vi "Execute.vi"(8 "error in":errorcluster, 11 "O3 Power On in":refnum<class "O3 Power On.lvclass">) -> (0 "error out":errorcluster, 1 "Next Step?":bool, 2 "MSG":string, 3 "O3 Power On out":refnum<class "O3 Power On.lvclass">)   [LabVIEW 2015, in "O3 Power On.lvclass"]
uses:
  O3 Power On.lvclass
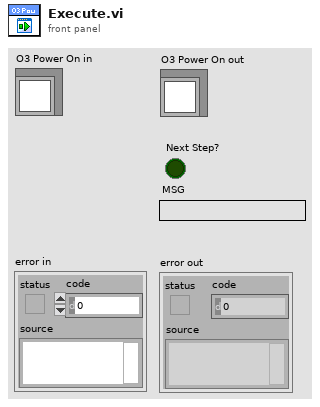
[diagram p1: front panel]
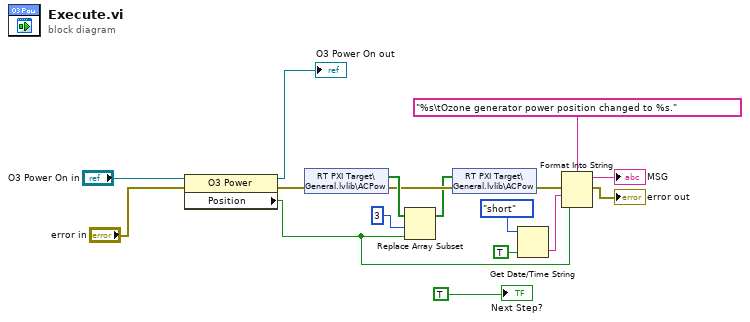
[diagram p0: block diagram]
diagram:
  n1 = property class="O3 Power"(reference="O3 Power On in", error in="error in") -> (reference out=→"O3 Power On out":refnum<class "O3 Power On.lvclass">, error out=w4:errorcluster, "Position"=w1:bool)
  n2 = shared-variable "RT PXI Target\\General.lvlib\\ACPow"(error in=w4) -> (w6:bool[], error out=w3:errorcluster)
  n3 = Replace Array Subset(array=w6, new element=w1, index=3) -> (w2:bool[])
  n4 = shared-variable "RT PXI Target\\General.lvlib\\ACPow"(w2, error in=w3) -> (error out=w13:errorcluster)
  n5 = Get Date/Time String(date format (0)=enum16{"short", "long", "abbreviated"}."short", want seconds? (F)=TRUE) -> (time string=w15:string)  [unwired: 1 in, 1 out]
  n6 = Format Into String(format string="%s\tOzone generator power position changed to %s.", error in=w13, w15, w1) -> (resulting string=→"MSG":string, error out=→"error out":errorcluster)  [unwired: 1 in]
  "Next Step?" <- TRUE ("Next Step?")
